vi "Get Experiment Statuses.vi"(8 "error in (no error)":errorcluster, 11 "eLab in":refnum<class "PL eLabFTW Client.lvclass">) -> (0 "error out":errorcluster, 2 "statuses":T1(array[cluster]), 3 "eLab out":refnum<class "PL eLabFTW Client.lvclass">)   [LabVIEW 2015, in "PL eLabFTW Client.lvclass"]
doc: "Gets experiment statuses."
uses:
  PL eLabFTW Client.lvclass
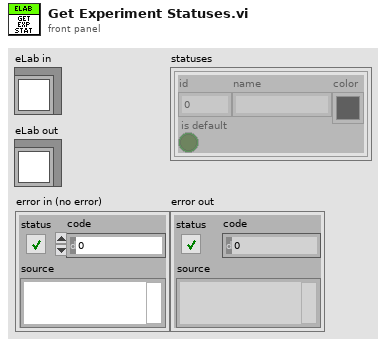
[diagram p1: front panel]
types:
  T1 = cluster{"id":u32, "name":string, "color":u32, "is default":bool}[]
  T2 = cluster{"category_id":string, "category":string, "color":string, "is_default":string}[]
  T3 = cluster{"id":u32, "name":string, "color":u32, "is default":bool}
  T4 = cluster{"category_id":i32, "category":i32, "color":i32, "is_default":i32}
  T5 = cluster{"category_id":bool, "category":bool, "color":bool, "is_default":bool}
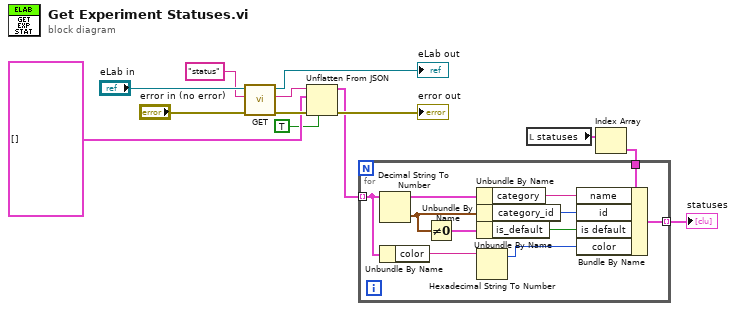
[diagram p0: block diagram]
diagram:
  n1 = call "GET.vi"("error in (no error)"="error in (no error)", "relative URL"="status", "eLab in"="eLab in") -> ("error out"=w8:errorcluster, "response body"=w9:string, "eLab out"=→"eLab out":refnum<class "PL eLabFTW Client.lvclass">)  [unwired: 6 in]
  n2 = Unflatten From JSON(JSON string=w9, type and defaults=T2 [], default null elements? (F)=TRUE, error in (no error)=w8) -> (value=w5:T2, error out=→"error out":errorcluster)  [unwired: 3 in]
  n3 = local read "statuses"() -> (w4:T1)
  n4 = Index Array(array=w4) -> (element=w3:T3)  [unwired: 1 in]
  n5 = for {
    tunnel: w5 -> [w17] mode=indexing
    tunnel: w3 -> [w14]
    tunnel: [w23] -> w2 mode=indexing
    n6 = Decimal String To Number(string=w17) -> (number=w21:T4)  [unwired: 2 in, 1 out]
    n7 = Unbundle By Name(w17) -> ("color"=w16:string)
    n8 = Not Equal To 0?(x=w21) -> (x != 0?=w20:T5)
    n9 = Unbundle By Name(w17) -> ("category"=w22:string)
    n10 = Unbundle By Name(w21) -> ("category_id"=w19:i32)
    n11 = Unbundle By Name(w20) -> ("is_default"=w18:bool)
    n12 = Hexadecimal String To Number(string=w16) -> (offset past number=w15:i32)  [unwired: 2 in, 1 out]
    n13 = Bundle By Name(cluster=w14, "name"=w22, "id"=w19, "is default"=w18, "color"=w15) -> (w23:T3)
  }
  "statuses" <- w2
